vi "Trapezoidal State Handler.vi"(6 "Reset?":bool, 8 "Current State":T1, 9 "Current Time":dbl, 10 "Time per State":dbl[](array[numeric]), 11 "Upcoming States":T1[](array[typedef])) -> (1 "Time Left":dbl, 3 "New State":T1, 5 "State Time":dbl)   [LabVIEW 2015]
uses:
  Trapezoidal Motion State.ctl
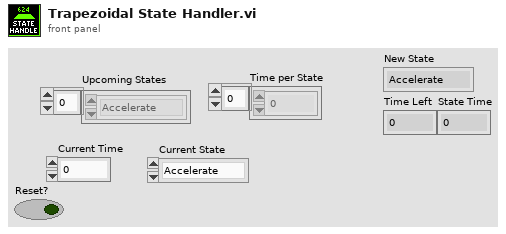
[diagram p1: front panel]
types:
  T1 = typedef "Trapezoidal Motion State.ctl" = enum16{"Accelerate", "Cruise", "Decelerate", "Finish"}
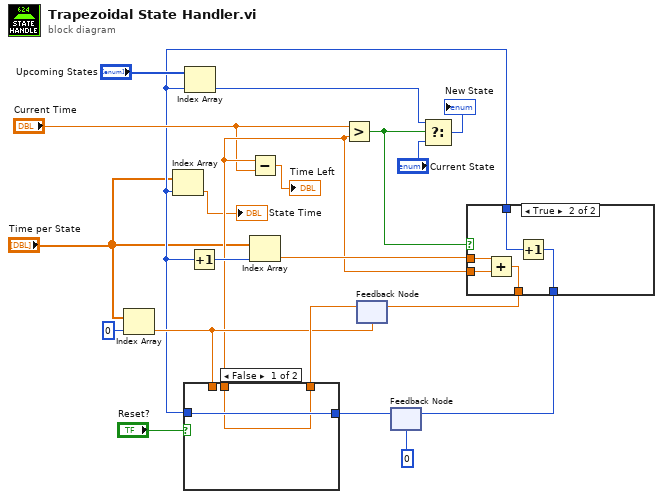
[diagram p0: block diagram]
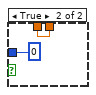
[diagram p2: hidden frame]
diagram:
  n1 = Index Array(array="Time per State", index=0) -> (element=w8:dbl)
  n2 = feedback #1(w8) -> (w12:dbl)
  n3 = feedback #2(0) -> (w14:i32)
  n4 = case shown="False" "Reset?" {
    tunnel: w14 -> [w23 _]
    tunnel: [w23 0] -> w3
    tunnel: w12 -> [w22 _]
    tunnel: [w22 w24] -> w6
    tunnel: w8 -> [_ w24]
    frame False {
    }
    frame True {
    }
  }
  n5 = Index Array(array="Time per State", index=w3) -> (element=→"State Time":dbl)
  n6 = Index Array(array="Upcoming States", index=w3) -> (element=w18:T1)
  n7 = Increment(x=w3) -> (x+1=w7:i32)
  n8 = Subtract(x=w6, y="Current Time") -> (x-y=→"Time Left":dbl)
  n9 = Index Array(array="Time per State", index=w7) -> (element=w11:dbl)
  n10 = Greater?(x="Current Time", y=w6) -> (0:w16:bool)
  n11 = Select(t=w18, s=w16, f="Current State") -> (s? t:f=→"New State":T1)
  n12 = case shown="True" w16 {
    tunnel: w3 -> [w27 w32]
    tunnel: [w27 w31] -> w15
    tunnel: w11 -> [_ w30]
    tunnel: [w26 w29] -> w10
    tunnel: w6 -> [w26 w28]
    frame False {
    }
    frame True {
      n13 = Add(x=w30, y=w28) -> (x+y=w29:dbl)
      n14 = Increment(x=w32) -> (x+1=w31:i32)
    }
  }
  n15 = feedback-in #1(w10) -> ()
  n16 = feedback-in #2(w15) -> ()
